vi "$CTL_PumpCtlr.vi"(8 "Pump Manual Controls":T2={"Pump Speed"=enum."STOP", "FILL"=FALSE, "Drain"=FALSE, "Auto/!Man"=TRUE, "Sim Level"=TRUE, "Raw Leve/\n!Level PVl"=TRUE, "Jog"=FALSE}, 9 "Pump Params":T1={"Empty Inches"=8.0, "Full Inches"=2.5, "RNG_SLOW"=0.5, "RNG_CREEP"=0.007, "RNG_STOP "=0.002, "VISA resource name"="COM4", "SPD_SLOW"=30, "SPD_CREEP"=7, "SPD_FAST"=100, "Zero template"=path "C:/AllenProjects/PWC-OLS/$Calibrtation/CAL_Level_RnR_241105.xlsx", "zero  Settle sec"=5, "Laser Slope"=-0.996, "Laser Offset"=9.601, "Sim Fill Rate"=0.0, "Cal Date"="", "Cal Technician"=""} {"Sim Fill Rate" format="%.3f"; "Laser Offset" format="%.3f"; "Laser Slope" format="%.3f"; "RNG_STOP" format="%#_13g"; "RNG_CREEP" format="%#_13g"; "RNG_SLOW" format="%#_13g"}, 10 "Level PV":dbl=8.1, 11 "Level SP":dbl=8.0) -> (1 "Pump Speed Out":T3=enum."STOP", 2 "X< Neg":bool, 3 "X>Pos":bool, 5 "Neg <X<Pos":bool=TRUE)   [LabVIEW 2024]
uses:
  Control Definitions/Def_PumpSpeed.ctl
  Control Definitions/DEF_PumpManCtl.ctl
  Control Definitions/DEF_PumpParams.ctl
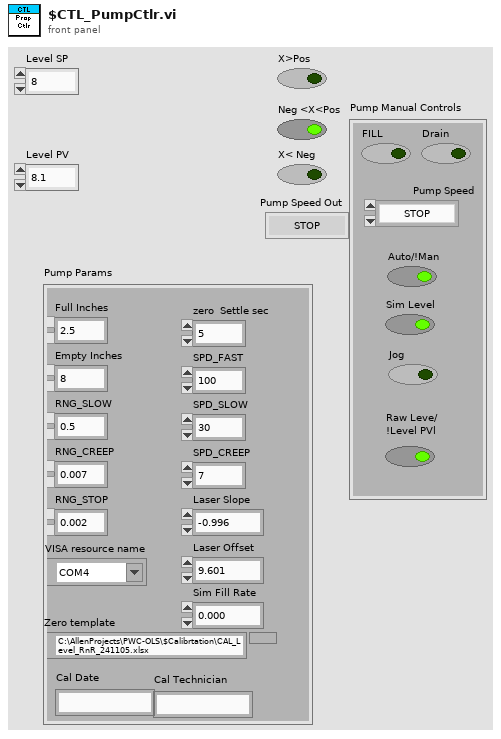
[diagram p1: front panel]
types:
  T1 = typedef "DEF_PumpParams.ctl" = cluster{"Empty Inches":dbl, "Full Inches":dbl, "RNG_SLOW":dbl, "RNG_CREEP":dbl, "RNG_STOP ":dbl, "VISA resource name":refnum<visa-resource-name>, "SPD_SLOW":i32, "SPD_CREEP":i32, "SPD_FAST":i32, "Zero template":path, "zero  Settle sec":i32, "Laser Slope":sgl, "Laser Offset":sgl, "Sim Fill Rate":sgl, "Cal Date":string, "Cal Technician":string}
  T2 = typedef "DEF_PumpManCtl.ctl" = cluster{"Pump Speed":T3, "FILL":bool, "Drain":bool, "Auto/!Man":bool, "Sim Level":bool, "Raw Leve/\n!Level PVl":bool, "Jog":bool}
  T3 = typedef "Def_PumpSpeed.ctl" = enum16{"FAST", "SLOW", "CREEP", "STOP"}
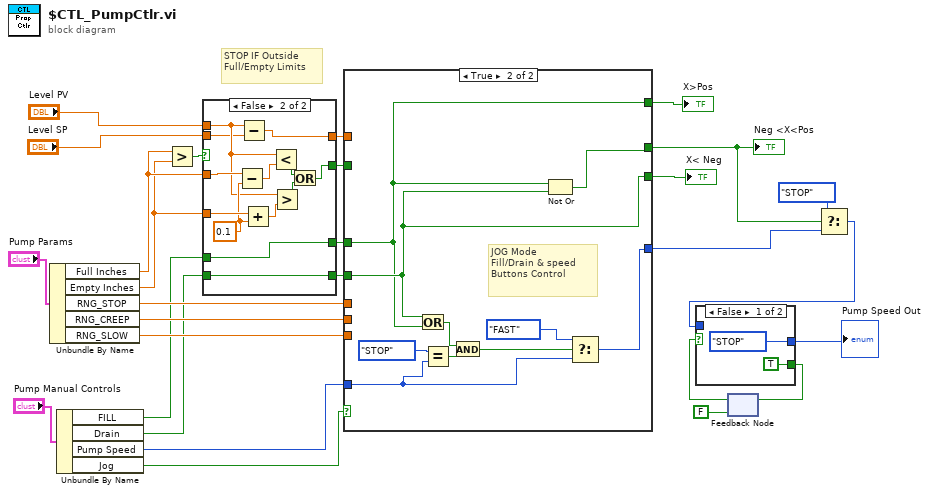
[diagram p0: block diagram]
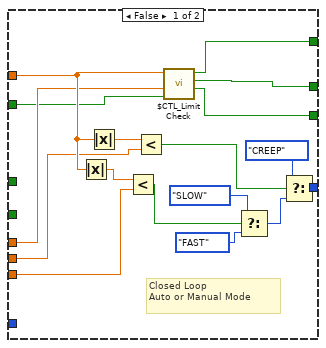
[diagram p2: hidden frame]
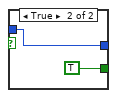
[diagram p3: hidden frame]
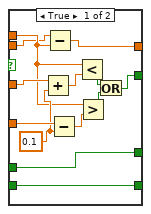
[diagram p4: hidden frame]
diagram:
  # "STOP IF Outside\nFull/Empty Limits"
  n1 = Unbundle By Name("Pump Params") -> ("Full Inches"=w12:dbl, "Empty Inches"=w11:dbl, "RNG_STOP"=w13:dbl, "RNG_CREEP"=w14:dbl, "RNG_SLOW"=w15:dbl)
  n2 = Unbundle By Name("Pump Manual Controls") -> ("FILL"=w5:bool, "Drain"=w3:bool, "Pump Speed"=w6:T3, "Jog"=w7:bool)
  n3 = Greater?(x=w12, y=w11) -> (0:w16:bool)
  n4 = case shown="False" w16 {
    tunnel: [w41 w54] -> w24
    tunnel: "Level PV" -> [w30 w43]
    tunnel: "Level SP" -> [w29 w42]
    tunnel: w12 -> [w34 w47]
    tunnel: w11 -> [w37 w50]
    tunnel: [w38 w51] -> w9
    tunnel: w5 -> [w32 w45]
    tunnel: [w32 w45] -> w4
    tunnel: w3 -> [w31 w44]
    tunnel: [w31 w44] -> w2
    frame True {
      w33 = 0.1 ("y")
      n5 = Add(x=w34, y=w33) -> (x+y=w35:dbl)
      n6 = Subtract(x=w29, y=w30) -> (x-y=w41:dbl)
      n7 = Subtract(x=w37, y=w33) -> (x-y=w36:dbl)
      n8 = Less?(x=w30, y=w35) -> (x < y?=w39:bool)
      n9 = Greater?(x=w30, y=w36) -> (0:w40:bool)
      n10 = Or(x=w39, y=w40) -> (x .or. y?=w38:bool)
    }
    frame False {
      w46 = 0.1 ("y")
      n11 = Subtract(x=w47, y=w46) -> (x-y=w48:dbl)
      n12 = Subtract(x=w43, y=w42) -> (x-y=w54:dbl)
      n13 = Add(x=w50, y=w46) -> (x+y=w49:dbl)
      n14 = Less?(x=w43, y=w48) -> (x < y?=w52:bool)
      n15 = Greater?(x=w43, y=w49) -> (0:w53:bool)
      n16 = Or(x=w52, y=w53) -> (x .or. y?=w51:bool)
    }
  }
  n17 = case shown="True" w7 {
    tunnel: [w69 w78] -> w28
    tunnel: [w68 w79] -> w25
    tunnel: w24 -> [w64 _]
    tunnel: [w60 w73] -> w22
    tunnel: w15 -> [w59 _]
    tunnel: w14 -> [w58 _]
    tunnel: w13 -> [w57 _]
    tunnel: [w56 w81] -> w10
    tunnel: w9 -> [w55 _]
    tunnel: w6 -> [_ w74]
    tunnel: w4 -> [_ w78]
    tunnel: w2 -> [_ w79]
    frame False {
      # "Closed Loop\nAuto or Manual Mode"
      n18 = Absolute Value(x=w64) -> (abs(x)=w70:dbl)
      n19 = Absolute Value(x=w64) -> (abs(x)=w65:dbl)
      n20 = Less?(x=w70, y=w59) -> (x < y?=w71:bool)
      n21 = Less?(x=w65, y=w58) -> (x < y?=w67:bool)
      n22 = call "$CTL_Limit Check.vi"("E-Stop"=w55, "Limit"=w57, "X"=w64) -> ("X< Neg"=w68:bool, "Neg <X<Pos"=w56:bool, "X>Pos"=w69:bool)  [unwired: 6 in]
      n23 = Select(t=Def_PumpSpeed."SLOW" ("Pump Speed"), s=w71, f=Def_PumpSpeed."FAST") -> (s? t:f=w62:T3)
      n24 = Select(t=Def_PumpSpeed."CREEP" ("Pump Speed"), s=w67, f=w62) -> (s? t:f=w60:T3)
    }
    frame True {
      # "JOG Mode\nFill/Drain & speed\nButtons Control"
      n25 = Or(x=w79, y=w78) -> (x .or. y?=w76:bool)
      n26 = Equal?(x=Def_PumpSpeed."STOP", y=w74) -> (x = y?=w77:bool)
      n27 = And(x=w76, y=w77) -> (x .and. y?=w75:bool)
      n28 = Not Or(1:w79, 2:w78) -> (0:w81:bool)
      n29 = Select(t=Def_PumpSpeed."FAST", s=w75, f=w74) -> (s? t:f=w73:T3)
    }
  }
  "X>Pos" <- w28
  "X< Neg" <- w25
  "Neg <X<Pos" <- w10
  n30 = feedback #1(FALSE) -> (w21:bool)
  n31 = Select(t=Def_PumpSpeed."STOP" ("Pump Speed"), s=w10, f=w22) -> (s? t:f=w17:T3)
  n32 = case shown="False" w21 {
    tunnel: [TRUE TRUE] -> w20
    tunnel: [Def_PumpSpeed."STOP" ("Pump Speed") w84] -> w18
    tunnel: w17 -> [_ w84]
    frame False {
    }
    frame True {
    }
  }
  "Pump Speed Out" <- w18
  n33 = feedback-in #1(w20) -> ()
